vi "ADC.vi"() -> (3 "Output":u32)   [LabVIEW 2009]
doc: "Loops indefinetly awaiting a Run confirmation. Disables other devices and performs a new conversion every second. The result of every conversion is a 32 bit code."
uses:
  <vilib>/eio/EIONode/EIONode.xnode
  <vilib>/rvi/eio/nirviEIOImplementation/nirviEIOImplementation.xnode
  <vilib>/rvi/eio/common/nirviEmuTemplateMethod_noerrors.vi
  <vilib>/rvi/eio/common/nirviEmuClasses.ctl
  Instance           5 11Saved   ADC .vi
  Instance           4 11Saved   ADC .vi
  Instance           3 11Saved   ADC .vi
  Instance           2 11Saved   ADC .vi
  Instance           1 11Saved   ADC .vi
panel:
  # "Use ADChost.vi to control this FPGA VI"
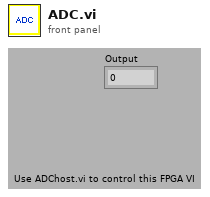
[diagram p1: front panel]
types:
  T1 = typedef "nirviEmuClasses.ctl" = enum16{"IO Read", "IO Write", "Method", "Property Read", "Property Write"}
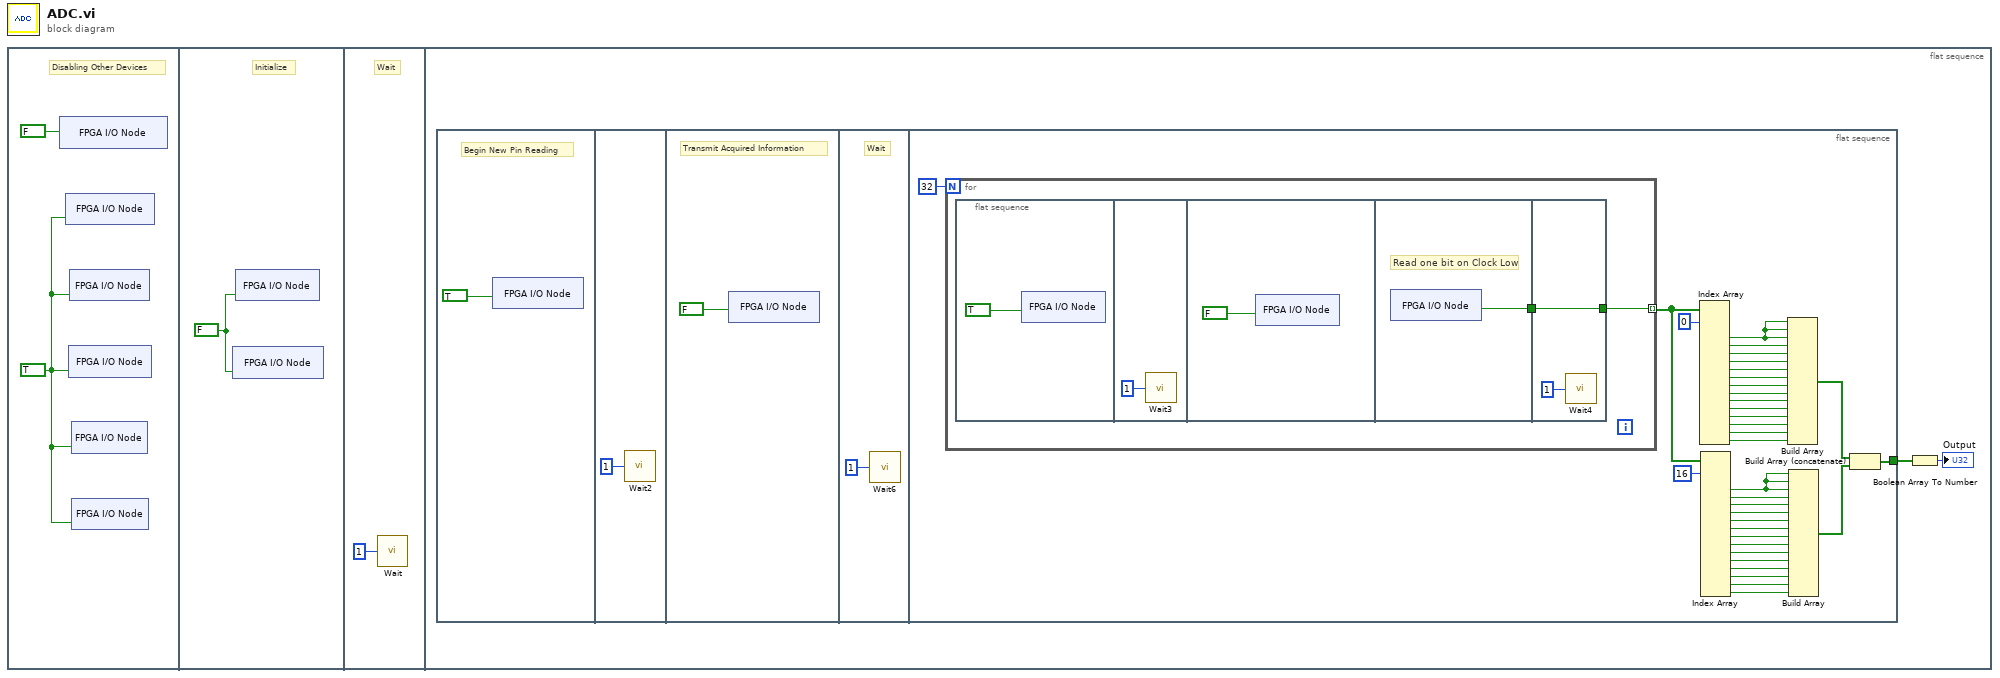
[diagram p0: block diagram]
diagram:
  n1 = flat-sequence {
    frame #0 {
      w2 = TRUE
      # "Disabling Other Devices"
      n2 = xnode "FPGA I/O Node"("FPGA_INIT_B"=FALSE) -> ()  [unwired: 1 in, 1 out]
      n3 = xnode "FPGA I/O Node"("SPI_SS_B"=w2) -> ()  [unwired: 1 in, 1 out]
      n4 = xnode "FPGA I/O Node"("DAC_CS"=w2) -> ()  [unwired: 1 in, 1 out]
      n5 = xnode "FPGA I/O Node"("SF_CE0"=w2) -> ()  [unwired: 1 in, 1 out]
      n6 = xnode "FPGA I/O Node"("SF_OE"=w2) -> ()  [unwired: 1 in, 1 out]
      n7 = xnode "FPGA I/O Node"("SF_WE"=w2) -> ()  [unwired: 1 in, 1 out]
    }
    frame #1 {
      w75 = FALSE ("SPI_SCK")
      # "Initialize"
      n8 = xnode "FPGA I/O Node"("AD_CONV"=w75) -> ()  [unwired: 1 in, 1 out]
      n9 = xnode "FPGA I/O Node"("SPI_SCK"=w75) -> ()  [unwired: 1 in, 1 out]
    }
    frame #2 {
      # "Wait"
      n10 = call "Wait"("Count(Ticks)"=u32 1) -> ()  [unwired: 1 out]
    }
    frame #3 {
      n11 = flat-sequence {
        tunnel: [w131] -> w101
        frame #0 {
          # "Begin New Pin Reading"
          n12 = xnode "FPGA I/O Node"("AD_CONV"=TRUE) -> ()  [unwired: 1 in, 1 out]
        }
        frame #1 {
          n13 = call "Wait2"("Count(Ticks)"=u32 1) -> ()  [unwired: 1 out]
        }
        frame #2 {
          # "Transmit Acquired Information"
          n14 = xnode "FPGA I/O Node"("AD_CONV"=FALSE) -> ()  [unwired: 1 in, 1 out]
        }
        frame #3 {
          # "Wait"
          n15 = call "Wait6"("Count(Ticks)"=u32 1) -> ()  [unwired: 1 out]
        }
        frame #4 {
          n16 = for {
            N: 32 -> [_]
            tunnel: [w166] -> w136 mode=indexing
            n17 = flat-sequence {
              tunnel: [w195] -> w167
              tunnel: [w216] -> w166
              tunnel: w167 -> [w216]
              frame #0 {
                n18 = xnode "FPGA I/O Node"("SPI_SCK"=TRUE) -> ()  [unwired: 1 in, 1 out]
              }
              frame #1 {
                n19 = call "Wait3"("Count(Ticks)"=u32 1) -> ()  [unwired: 1 out]
              }
              frame #2 {
                n20 = xnode "FPGA I/O Node"("SPI_SCK"=FALSE) -> ()  [unwired: 1 in, 1 out]
              }
              frame #3 {
                # "Read one bit on Clock Low"
                n21 = xnode "FPGA I/O Node"() -> ("SPI_MISO"=w195:bool)  [unwired: 1 in, 1 out]
              }
              frame #4 {
                n22 = call "Wait4"("Count(Ticks)"=u32 1) -> ()  [unwired: 1 out]
              }
            }
          }
          n23 = Index Array(array=w136, index #1=0 ("index")) -> (element #3=w151:bool, element #4=w164:bool, element #5=w163:bool, element #6=w162:bool, element #7=w161:bool, element #8=w160:bool, element #9=w159:bool, element #10=w158:bool, element #11=w157:bool, element #12=w156:bool, element #13=w155:bool, element #14=w154:bool, element #15=w153:bool, element #16=w152:bool)  [unwired: 15 in, 2 out]
          n24 = Index Array(array=w136, index #1=16 ("index")) -> (element #3=w150:bool, element #4=w137:bool, element #5=w138:bool, element #6=w139:bool, element #7=w140:bool, element #8=w141:bool, element #9=w142:bool, element #10=w143:bool, element #11=w144:bool, element #12=w145:bool, element #13=w146:bool, element #14=w147:bool, element #15=w148:bool, element #16=w149:bool)  [unwired: 15 in, 2 out]
          n25 = Build Array(w151, w151, w151, w164, w163, w162, w161, w160, w159, w158, w157, w156, w155, w154, w153, w152) -> (w133:bool[])
          n26 = Build Array(w150, w150, w150, w137, w138, w139, w140, w141, w142, w143, w144, w145, w146, w147, w148, w149) -> (w132:bool[])
          n27 = Build Array (concatenate)(w133, w132) -> (w131:bool[])
        }
      }
      n28 = Boolean Array To Number(Boolean array=w101) -> (number=→"Output":u32)
    }
  }
